vi "DataBase Queue - Enqueue.vi"(6 "Priority Message? (F)":bool, 8 "error in":errorcluster, 10 "Value":variant, 11 "Message":string) -> (0 "error out":errorcluster)   [LabVIEW 2024, in "Data Base.lvlib"]
uses:
  Data Base.lvlib
  Support/General Type Defs/FGV States.ctl
  Support/QMH Messaging/QMH - Enqueue Element.vi
  Support/General Type Defs/General Type Defs.lvlib
  Support/QMH Messaging/QMH Messaging.lvlib
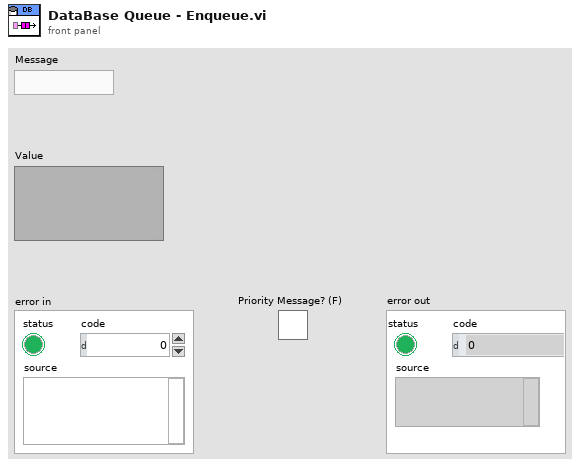
[diagram p1: front panel]
types:
  T1 = typedef "General Type Defs.lvlib/FGV States.ctl" = enum16{"Create", "Get", "Destroy"}
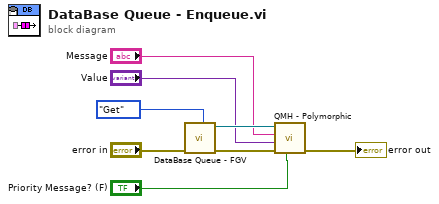
[diagram p0: block diagram]
diagram:
  n1 = call "DataBase Queue - FGV.vi"("FGV States"=FGV_States."Get", "error in"="error in") -> ("error out"=w5:errorcluster, "queue out"=w6:refnum<queue>)  [unwired: 8 in]
  n2 = call-poly "QMH - Polymorphic.vi"("Priority Message? (F)"="Priority Message? (F)", "error in (no error)"=w5, "Message Data"="Value", "Message"="Message", "Message Queue"=w6) -> ("error out"=→"error out":errorcluster)  [unwired: 5 in, 1 out]
